vi "Record Call.vi"(8 "error in (no error)":errorcluster, 10 "VI Call":refnum<class "VI Call.lvclass">, 11 "One In":refnum<class "One.lvclass">) -> (0 "error out":errorcluster, 3 "One Out":refnum<class "One.lvclass">)   [LabVIEW 2020, in "One.lvclass"]
uses:
  One.lvclass
  Framework/VI Call/VI Call.lvclass
  One.lvclass/One.ctl
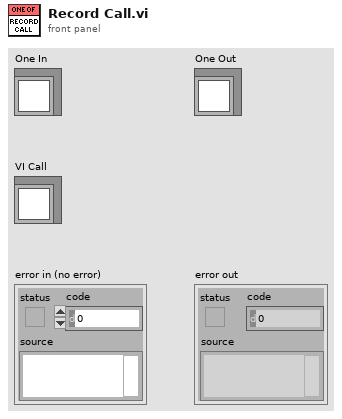
[diagram p1: front panel]
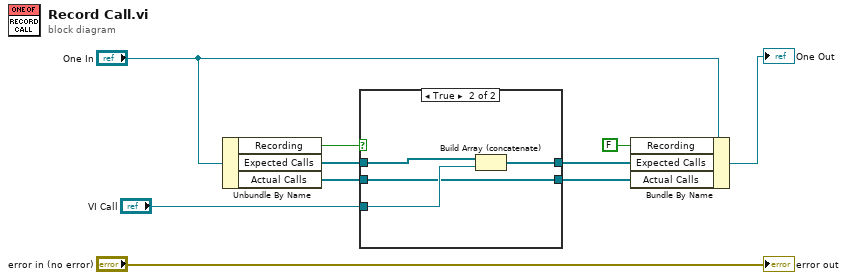
[diagram p0: block diagram]
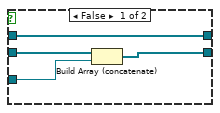
[diagram p2: hidden frame]
diagram:
  n1 = Unbundle By Name("One In") -> ("Recording"=w7:bool, "Expected Calls"=w4:refnum<class "VI Call.lvclass">[], "Actual Calls"=w2:refnum<class "VI Call.lvclass">[])
  n2 = case shown="True" w7 {
    tunnel: "VI Call" -> [w13 w17]
    tunnel: w4 -> [w12 w18]
    tunnel: [w12 w16] -> w3
    tunnel: w2 -> [w14 w15]
    tunnel: [w11 w15] -> w1
    frame False {
      n3 = Build Array (concatenate)(w14, w13) -> (w11:refnum<class "VI Call.lvclass">[])
    }
    frame True {
      n4 = Build Array (concatenate)(w18, w17) -> (w16:refnum<class "VI Call.lvclass">[])
    }
  }
  n5 = Bundle By Name(cluster="One In", "Recording"=FALSE, "Expected Calls"=w3, "Actual Calls"=w1) -> (→"One Out":refnum<class "One.lvclass">)
  "error out" <- "error in (no error)"
